vi "Z900_navX_ProcessingLoop.vi"(11 "navX Device":T1={"Interface"={"Protocol"=enum."SERIAL", "Update Rate (4Hz-60Hz)"=4, "navX Open TypeDef"=variant}, "Notify Packet"=refnum, "Loop VI Refnum"=refnum} {"Interface"."Update Rate (4Hz-60Hz)" min=4 max=60 step=1}) -> (2 "Local Registry":u8[](array[numeric]))   [LabVIEW 2014, in "navX Library v2.lvlib"]
uses:
  navX Library v2.lvlib
  TypeDefs/Z900_navX_DeviceTypeDef.ctl
  TypeDefs/Z900_navX_ProtocolTypeDef.ctl
  TypeDefs/Z900_navX_NotifyPacketTypeDef.ctl
  TypeDefs/Z900_navX_ActionTypeDef.ctl
  <vilib>/Platform/TimedLoop/XDataNode/timing_clust.ctl
  <vilib>/Platform/TimedLoop/XDataNode/nitl_modes.ctl
  <vilib>/Platform/TimedLoop/XDataNode/wakeup.ctl
  <vilib>/Rock Robotics/SystemInterfaces/Utilities/FPGA_UtilitiesRead LocalTime.vi
  <vilib>/platform/TimedLoop/XDataNode/XDataNode.xnode
  <vilib>/Platform/TimedLoop/XDataNode/XDNodeRunTimeDep.lvlib
panel:
  in  "Halt":bool
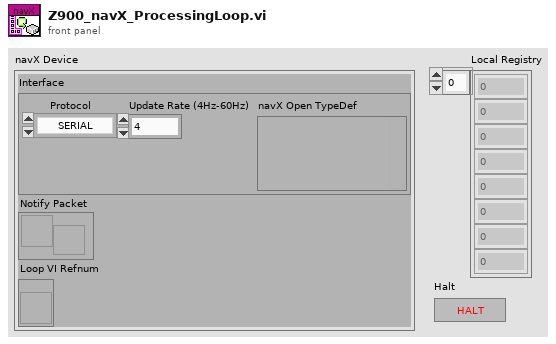
[diagram p1: front panel]
types:
  T1 = typedef "navX Library v2.lvlib/Z900_navX_DeviceTypeDef.ctl" = cluster{"Interface":cluster{"Protocol":T2, "Update Rate (4Hz-60Hz)":u8, "navX Open TypeDef":variant}, "Notify Packet":refnum<notifier>, "Loop VI Refnum":refnum<vi>}
  T2 = typedef "navX Library v2.lvlib/Z900_navX_ProtocolTypeDef.ctl" = enum16{"SERIAL", "I2C", "SPI"}
  T3 = cluster{"Last Valid FPGA Time":dbl, "Error Count":i32, "Initialized":bool}
  T4 = typedef "navX Library v2.lvlib/Z900_navX_InterfaceTypeDef.ctl" = cluster{"SerialPortRef":T5, "I2CDevRef":T6, "SPIDevRef":T9}
  T5 = typedef "WPI_SerialPortRef.ctl" = cluster{"DevStatus":errorcluster, "Serial Port Name":refnum<visa-resource-name>}
  T6 = typedef "WPI_I2CDevRef.ctl" = cluster{"DevStatus":errorcluster, "Controller":T7, "Device Address":u8, "Handle":i32, "I2C Bus":T8}
  T7 = typedef "FPGA_TypedefDigitalModule.ctl" = enum16{"Controller 1"}
  T8 = typedef "i2c_bus.ctl" = enum16{"I2C On-Board", "I2C MXP", "Invalid"}
  T9 = typedef "WPI_SPIDevRef.ctl" = cluster{"DevStatus":errorcluster, "Handle":i32, "Controller":T7, "SPI Bus":T10}
  T10 = typedef "spi_bus.ctl" = enum16{"SPI On-Board, CS0", "SPI On-Board, CS1", "SPI On-Board, CS2", "SPI On-Board, CS3", "SPI MXP", "Invalid"}
  T11 = typedef "XDNodeRunTimeDep.lvlib/timing_clust.ctl" = cluster{"Expected End [f-1]":u64, "Actual End [f-1]":u64, "Finished Late? [f-1]":bool, "Expected End [i-1]":u64, "Actual End [i-1]":u64, "Finished Late? [i-1]":bool, "Expected Start [i]":u64, "Actual Start [i]":u64, "Expected Start [f]":u64, "Actual Start [f]":u64, "Source Name":string, "Structure Name":string, "Period":i64, "Deadline":i64, "Offset":i64, "Start":i64, "Priority":i32, "Timeout":i32, "Mode":T12, "Wakeup Reason":T13, "Error":errorcluster, "Source Type":string, "Secondary Source Type":string, "Global End Time":u64, "Global Start Time":u64, "Frame Duration":u64, "Iteration Duration":u64, "Assigned CPU":i32, "I/O Scan Engine Mode":u32}
  T12 = typedef "XDNodeRunTimeDep.lvlib/nitl_modes.ctl" = enum32{"No Change", "Process missed periods, maintain original phase", "Discard missed periods, maintain original phase", "Process missed periods, ignore original phase", "Discard missed periods, ignore original phase"}
  T13 = typedef "XDNodeRunTimeDep.lvlib/wakeup.ctl" = enum32{"Normal", "Aborted", "Asynchronous wakeup", "Timing source error", "Timed loop error", "Timeout"}
  T14 = typedef "navX Library v2.lvlib/Z900_navX_NotifyPacketTypeDef.ctl" = cluster{"navX Action":T15, "Data":variant}
  T15 = typedef "navX Library v2.lvlib/Z900_navX_ActionTypeDef.ctl" = enum16{"None", "Halt", "Reboot Detected", "Zero-Yaw"}
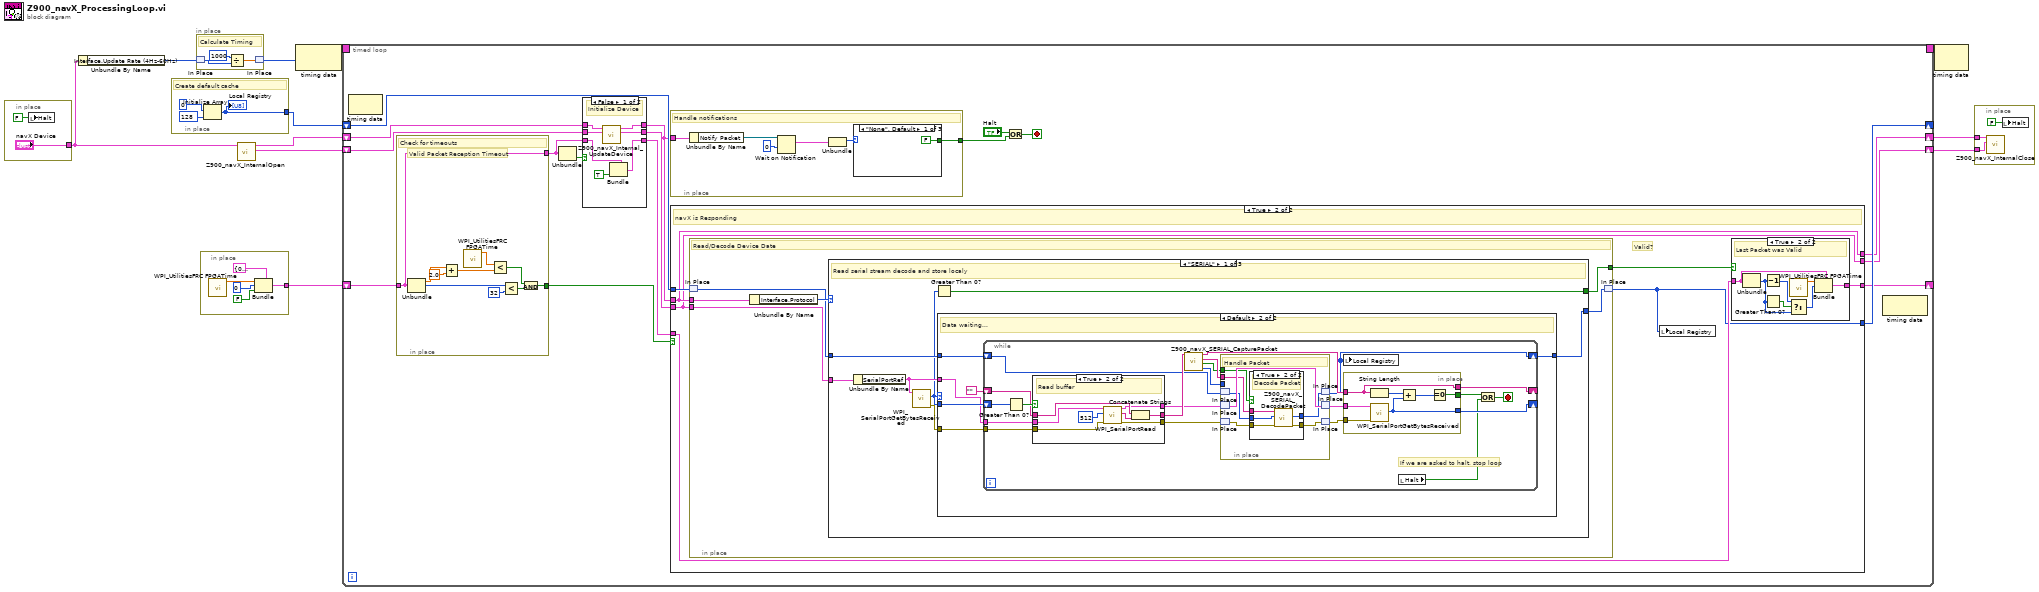
[diagram p0: block diagram]
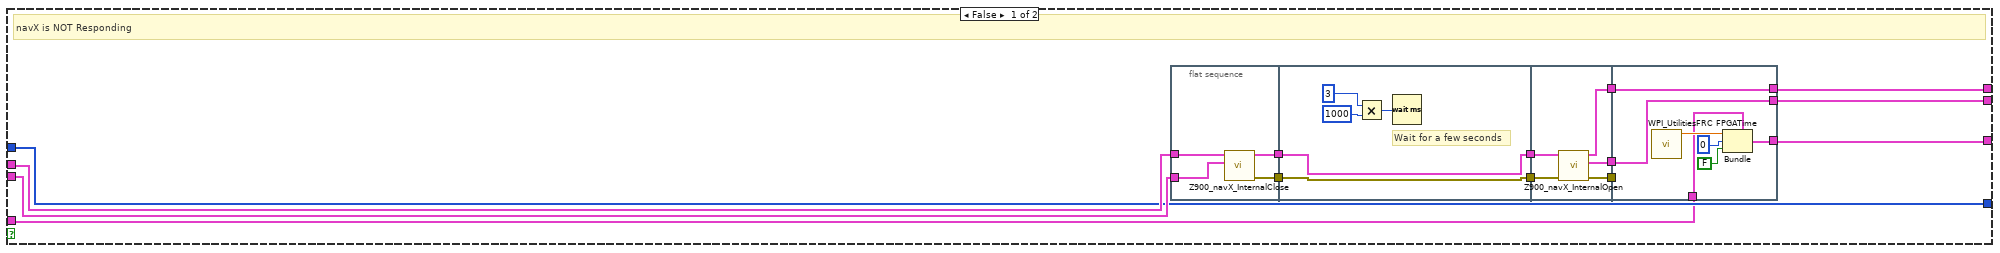
[diagram p3: hidden frame]
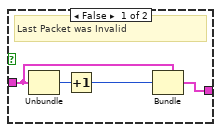
[diagram p4: hidden frame]
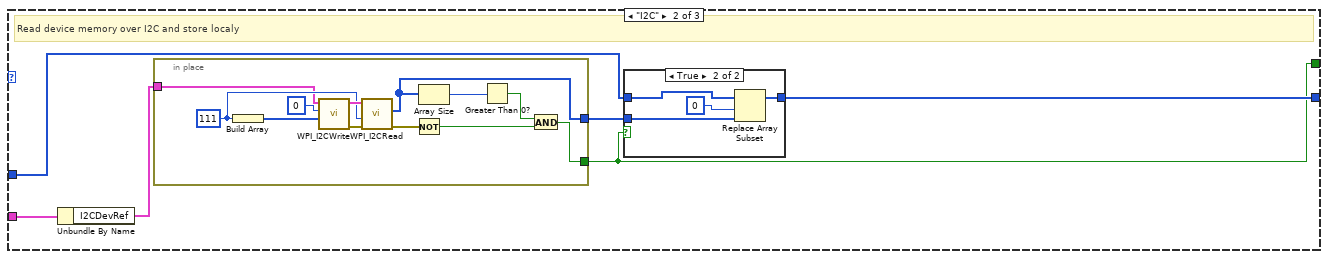
[diagram p8: hidden frame]
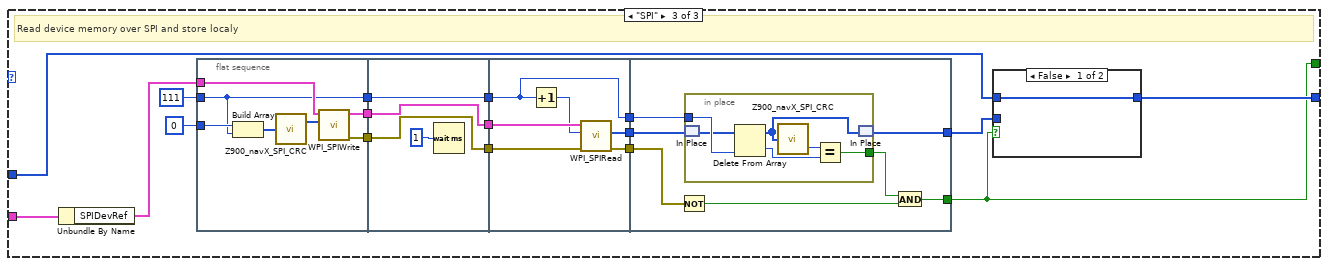
[diagram p10: hidden frame]
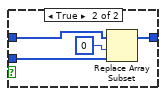
[diagram p11: hidden frame]
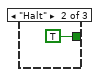
[diagram p12: hidden frame]
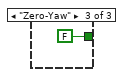
[diagram p13: hidden frame]
diagram:
  n1 = in-place {
    in-place-border: ["navX Device"] -> w4
    n2 = local write "Halt"(FALSE ("Halt")) -> ()
  }
  n3 = Unbundle By Name(w4) -> ("Interface.Update Rate (4Hz-60Hz)"=w8:u8)
  n4 = in-place {
    in-place-border: [w14] -> w7
    # "Create default cache"
    n5 = Initialize Array(u8 0 ("Received Data"), 128 ("hex")) -> (w14:u8[])
    "Local Registry" <- w14
  }
  n6 = in-place {
    # "Calculate Timing"
    n7 = in-place-match #1(w8) -> (w18:u8)
    n8 = Divide(x=1000, y=w18) -> (x/y=w17:dbl)
    n9 = in-place-match #1(w17) -> (w9:u8)
  }
  n10 = in-place {
    in-place-border: [w22] -> w2
    n11 = call <vilib>:"WPI_UtilitiesFRC FPGATime.vi"() -> ("FPGA Time"=w23:dbl)  [unwired: 10 in, 1 out]
    n12 = Bundle(cluster=T3 {"Last Valid FPGA Time"=0.0, "Error Count"=0, "Initialized"=FALSE}, "Last Valid FPGA Time"=w23, "Error Count"=0, "Initialized"=FALSE) -> (w22:T3)
  }
  n13 = call "Z900_navX_InternalOpen.vi"("navX Device"=w4) -> ("Interface TypeDefs"=w3:T4, "navX Device"=w1:T1)  [unwired: 8 in, 1 out]
  n14 = node-c288(w9) -> (w11:T11)
  n15 = timed-loop {
    timing: w11 -> [_]
    timing-out: [_] -> w10
    shift-right: [w40] -> _
    shift-left: w7 -> [w41]
    shift-right: [w34] -> w6
    shift-left: w1 -> [w31]
    shift-right: [w33] -> w5
    shift-left: w3 -> [w30]
    shift-right: [w39] -> _
    shift-left: w2 -> [w25]
    stop <- w36 stop-if-true
    n16 = node-c288() -> ()  [unwired: 1 in, 1 out]
    n17 = in-place {
      in-place-border: w25 -> [w52]
      in-place-border: [w53] -> w35
      in-place-border: [w52] -> w27
      # "Valid Packet Reception Timeout"
      # "Check for timeouts"
      n18 = Unbundle(w52) -> ("Last Valid FPGA Time"=w61:dbl, "Error Count"=w57:i32)  [unwired: 1 out]
      n19 = Add(x=w61, y=2.0) -> (x+y=w59:dbl)
      n20 = call <vilib>:"WPI_UtilitiesFRC FPGATime.vi"() -> ("FPGA Time"=w58:dbl)  [unwired: 10 in, 1 out]
      n21 = Less?(x=w58, y=w59) -> (x < y?=w55:bool)
      n22 = Less?(x=w57, y=32) -> (x < y?=w54:bool)
      n23 = And(x=w55, y=w54) -> (x .and. y?=w53:bool)
    }
    n24 = Unbundle(w27) -> ("Initialized"=w32:bool)  [unwired: 2 out]
    n25 = case shown="False" w32 {
      tunnel: w27 -> [w48 w51]
      tunnel: [w46 w51] -> w26
      tunnel: w31 -> [w45 w50]
      tunnel: w30 -> [w44 w49]
      tunnel: [w43 w50] -> w28
      tunnel: [w42 w49] -> w29
      frame False {
        # "Initialize Device"
        n26 = call "Z900_navX_Internal_UpdateDevice.vi"("Interface TypeDefs"=w44, "navX Device"=w45) -> ("Interface TypeDefs"=w42:T4, "navX Device"=w43:T1)  [unwired: 7 in, 1 out]
        n27 = Bundle(cluster=w48, "Initialized"=TRUE) -> (w46:T3)  [unwired: 2 in]
      }
      frame True {
      }
    }
    n28 = in-place {
      in-place-border: [w266] -> w38
      in-place-border: w28 -> [w265]
      # "Handle notifications"
      n29 = Unbundle By Name(w265) -> ("Notify Packet"=w264:refnum<notifier>)
      n30 = Wait on Notification(notifier=w264, timeout in ms (-1)=0) -> (notification=w268:T14)  [unwired: 2 in, 3 out]
      n31 = Unbundle(w268) -> ("navX Action"=w267:T15)  [unwired: 1 out]
      n32 = case shown="\"None\", Default" w267 {
        tunnel: [FALSE TRUE FALSE] -> w266
        frame "None", Default {
        }
        frame "Halt" {
        }
        frame "Zero-Yaw" {
        }
      }
    }
    n33 = case shown="True" w35 {
      tunnel: w41 -> [w73 w103]
      tunnel: w29 -> [w74 w100]
      tunnel: [w73 w97] -> w40
      tunnel: w26 -> [w63 w99]
      tunnel: [w62 w98] -> w39
      tunnel: w28 -> [w75 w101]
      tunnel: [w68 w101] -> w34
      tunnel: [w67 w100] -> w33
      frame False {
        # "navX is NOT Responding"
        n34 = flat-sequence {
          tunnel: w75 -> [w79]
          tunnel: w74 -> [w78]
          tunnel: [w77] -> w72
          tunnel: [w76] -> w71
          tunnel: w72 -> [w84]
          tunnel: w71 -> [w83]
          tunnel: [w84] -> w70
          tunnel: [w83] -> w69
          tunnel: w70 -> [w87]
          tunnel: w69 -> [w88]
          tunnel: [w89] -> w66
          tunnel: [w86] -> w65
          tunnel: [w85] -> w64
          tunnel: [w95] -> w67
          tunnel: [w96] -> w68
          tunnel: w66 -> [w96]
          tunnel: w65 -> [w95]
          tunnel: w64 -> [_]
          tunnel: w63 -> [w92]
          tunnel: [w91] -> w62
          frame #0 {
            n35 = call "Z900_navX_InternalClose.vi"("Interface TypeDefs"=w78, "navX Device"=w79) -> ("error out"=w77:errorcluster, "navX Device"=w76:T1)  [unwired: 8 in]
          }
          frame #1 {
            # "Wait for a few seconds"
            n36 = Multiply(x=u32 3 ("milliseconds to wait"), y=u32 1000) -> (x*y=w81:u32)
            n37 = Wait (ms)(milliseconds to wait=w81) -> ()  [unwired: 1 out]
          }
          frame #2 {
            n38 = call "Z900_navX_InternalOpen.vi"("error in"=w87, "navX Device"=w88) -> ("error out"=w85:errorcluster, "Interface TypeDefs"=w86:T4, "navX Device"=w89:T1)  [unwired: 7 in]
          }
          frame #3 {
            n39 = call <vilib>:"WPI_UtilitiesFRC FPGATime.vi"() -> ("FPGA Time"=w93:dbl)  [unwired: 10 in, 1 out]
            n40 = Bundle(cluster=w92, "Last Valid FPGA Time"=w93, "Error Count"=0, "Initialized"=FALSE) -> (w91:T3)
          }
        }
      }
      frame True {
        # "Valid?"
        # "navX is Responding"
        n41 = in-place {
          in-place-border: w101 -> [w115]
          in-place-border: w100 -> [w119]
          in-place-border: [w117] -> w102
          # "Read/Decode Device Date"
          n42 = in-place-match #2(w103) -> (w118:u8[])
          n43 = Unbundle By Name(w115) -> ("Interface.Protocol"=w120:T2)
          n44 = case shown="\"SERIAL\"" w120 {
            tunnel: [w125 w190 w218] -> w116
            tunnel: w118 -> [w126 w192 w227]
            tunnel: w119 -> [w127 w193 w226]
            tunnel: [w122 w189 w215] -> w117
            frame "SERIAL" {
              # "Read serial stream decode and store localy"
              n45 = Unbundle By Name(w127) -> ("SerialPortRef"=w123:T5)
              n46 = call <vilib>:"WPI_SerialPortGetBytesReceived.vi"("SerialPortRef"=w123) -> ("error out"=w124:errorcluster, "Bytes at Port"=w121:u32)  [unwired: 8 in, 1 out]
              n47 = Greater Than 0?(x=w121) -> (x > 0?=w122:bool)
              n48 = case shown="Default" w121 {
                tunnel: [w128 w134] -> w125
                tunnel: w126 -> [w128 w133]
                tunnel: w121 -> [_ w132]
                tunnel: w123 -> [_ w130]
                tunnel: w124 -> [_ w129]
                frame 0 {
                }
                frame Default {
                  # "Data waiting..."
                  n49 = while {
                    shift-right: [w135] -> w134
                    shift-left: w133 -> [w144]
                    shift-right: [w148] -> _
                    shift-left: w132 -> [w155]
                    shift-right: [w147] -> _
                    shift-left: "" -> [w153]
                    tunnel: w130 -> [w152]
                    tunnel: w129 -> [w151]
                    stop <- w138 stop-if-true
                    # "If we are asked to halt, stop loop"
                    n50 = Greater Than 0?(x=w155) -> (x > 0?=w154:bool)
                    n51 = case shown="True" w154 {
                      tunnel: w153 -> [w179 w187]
                      tunnel: w152 -> [w178 w186]
                      tunnel: w151 -> [w177 w183]
                      tunnel: [w179 w182] -> w150
                      tunnel: [w178 w181] -> w143
                      tunnel: [w177 w180] -> w142
                      frame False {
                        # "Pass existing buffer"
                      }
                      frame True {
                        # "Read buffer"
                        n52 = call <vilib>:"WPI_SerialPortRead.vi"("error in (no error)"=w183, "Num Bytes to Read"=u32 512, "SerialPortRef"=w186) -> ("error out"=w180:errorcluster, "Buffer"=w185:string, "SerialPortRef"=w181:T5)  [unwired: 6 in]
                        n53 = Concatenate Strings(w187, w185) -> (w182:string)
                      }
                    }
                    n54 = call "Z900_navX_SERIAL_CapturePacket.vi"("Buffer"=w150) -> ("Packet Size"=w145:i32, "Packet Located"=w136:bool, "Packet"=w146:string, "Buffer"=w149:string)  [unwired: 7 in]
                    n55 = in-place {
                      in-place-border: w146 -> [w160]
                      in-place-border: w136 -> [w161]
                      in-place-border: w145 -> [_]
                      # "Handle Packet"
                      n56 = in-place-match #3(w144) -> (w158:u8[])
                      n57 = in-place-match #4(w143) -> (w162:T5)
                      n58 = in-place-match #5(w142) -> (w157:errorcluster)
                      n59 = case shown="True" w161 {
                        tunnel: w160 -> [_ w169]
                        tunnel: [w164 w167] -> w159
                        tunnel: w158 -> [w164 w168]
                        tunnel: w157 -> [w163 w166]
                        tunnel: [w163 w165] -> w156
                        frame False {
                          # "No Packet"
                        }
                        frame True {
                          # "Decode Packet"
                          n60 = call "Z900_navX_SERIAL_DecodePacket.vi"("error in (no error)"=w166, "Data"=w168, "Packet"=w169) -> ("error out"=w165:errorcluster, "Data"=w167:u8[])  [unwired: 6 in, 1 out]
                        }
                      }
                      n61 = in-place-match #3(w159) -> (w135:u8[])
                      n62 = in-place-match #4(w162) -> (w140:T5)
                      n63 = in-place-match #5(w156) -> (w141:errorcluster)
                    }
                    n64 = local write "Local Registry"(w135) -> ()
                    n65 = in-place {
                      in-place-border: w140 -> [w176]
                      in-place-border: w141 -> [w175]
                      in-place-border: w149 -> [w170]
                      in-place-border: [w172] -> w139
                      in-place-border: [w171] -> w148
                      in-place-border: [w170] -> w147
                      n66 = String Length(string=w170) -> (length=w173:i32)
                      n67 = call <vilib>:"WPI_SerialPortGetBytesReceived.vi"("error in (no error)"=w175, "SerialPortRef"=w176) -> ("Bytes at Port"=w171:u32)  [unwired: 7 in, 2 out]
                      n68 = Add(x=w173, y=w171) -> (x+y=w174:u32)
                      n69 = Equal To 0?(x=w174) -> (x = 0?=w172:bool)
                    }
                    n70 = local read "Halt"() -> (w137:bool)
                    n71 = Or(x=w139, y=w137) -> (x .or. y?=w138:bool)
                  }
                }
              }
            }
            frame "I2C" {
              # "Read device memory over I2C and store localy"
              n72 = Unbundle By Name(w193) -> ("I2CDevRef"=w188:T6)
              n73 = in-place {
                in-place-border: [w197] -> w191
                in-place-border: [w196] -> w189
                in-place-border: w188 -> [w194]
                w202 = u8 111 ("hex")
                n74 = Build Array(w202) -> (w205:u8[])
                n75 = call <vilib>:"WPI_I2CWrite.vi"("I2CDataToSend"=w205, "I2CRegister"=u8 0 ("hex"), "I2CDevRef"=w194) -> ("error out"=w204:errorcluster, "I2CDevRef"=w203:T6)  [unwired: 7 in]
                n76 = call <vilib>:"WPI_I2CRead.vi"("error in (no error)"=w204, "I2CBytesToRead"=w202, "I2CDevRef"=w203) -> ("error out"=w198:errorcluster, "Data Out"=w197:u8[])  [unwired: 6 in, 1 out]
                n77 = Not(x=w198) -> (.not. x?=w195:bool)
                n78 = Array Size(array=w197) -> (size(s)=w200:i32)
                n79 = Greater Than 0?(x=w200) -> (x > 0?=w199:bool)
                n80 = And(x=w199, y=w195) -> (x .and. y?=w196:bool)
              }
              n81 = case shown="True" w189 {
                tunnel: w192 -> [w206 w210]
                tunnel: [w206 w209] -> w190
                tunnel: w191 -> [_ w208]
                frame False {
                }
                frame True {
                  n82 = Replace Array Subset(array=w210, new element=w208, index=u8 0 ("hex")) -> (w209:u8[])
                }
              }
            }
            frame "SPI" {
              # "Read device memory over SPI and store localy"
              n83 = Unbundle By Name(w226) -> ("SPIDevRef"=w211:T9)
              n84 = flat-sequence {
                tunnel: u8 0 ("hex") -> [w239]
                tunnel: u8 111 ("hex") -> [w234]
                tunnel: w211 -> [w236]
                tunnel: [w235] -> w224
                tunnel: [w234] -> w221
                tunnel: [w233] -> w214
                tunnel: w224 -> [w242]
                tunnel: [w242] -> w223
                tunnel: [w241] -> w222
                tunnel: w221 -> [w241]
                tunnel: w214 -> [w240]
                tunnel: [w240] -> w213
                tunnel: w223 -> [w249]
                tunnel: w222 -> [w246]
                tunnel: [w247] -> w220
                tunnel: [w246] -> w219
                tunnel: w213 -> [w245]
                tunnel: [w244] -> w212
                tunnel: w220 -> [w252]
                tunnel: w219 -> [w256]
                tunnel: [w253] -> w215
                tunnel: [w251] -> w217
                tunnel: w212 -> [w255]
                frame #0 {
                  n85 = Build Array(w239, w234) -> (w238:u8[])
                  n86 = call "Z900_navX_SPI_CRC.vi"("Message"=w238) -> ("Message with CRC"=w237:u8[])  [unwired: 1 out]
                  n87 = call <vilib>:"WPI_SPIWrite.vi"("Data To Send"=w237, "SPIDevRef"=w236) -> ("error out"=w233:errorcluster, "SPIDevRef"=w235:T9)  [unwired: 7 in, 1 out]
                }
                frame #1 {
                  n88 = Wait (ms)(milliseconds to wait=u32 1) -> ()  [unwired: 1 out]
                }
                frame #2 {
                  n89 = Increment(x=w246) -> (x+1=w248:u8)
                  n90 = call <vilib>:"WPI_SPIRead.vi"("error in (no error)"=w245, "Num to Read"=w248, "SPIDevRef"=w249) -> ("error out"=w244:errorcluster, "Received Data"=w247:u8[])  [unwired: 6 in, 1 out]
                }
                frame #3 {
                  n91 = Not(x=w255) -> (.not. x?=w250:bool)
                  n92 = in-place {
                    in-place-border: w256 -> [w262]
                    in-place-border: [w259] -> w254
                    n93 = in-place-match #6(w252) -> (w258:u8[])
                    n94 = Delete From Array(array=w258, index=w262) -> (deleted portion=w261:u8, array with subset deleted=w257:u8[])  [unwired: 1 in]
                    n95 = call "Z900_navX_SPI_CRC.vi"("Message"=w257) -> ("CRC"=w260:u8)  [unwired: 1 out]
                    n96 = Equal?(x=w260, y=w261) -> (x = y?=w259:bool)
                    n97 = in-place-match #6(w257) -> (w251:u8[])
                  }
                  n98 = And(x=w254, y=w250) -> (x .and. y?=w253:bool)
                }
              }
              n99 = case shown="False" w215 {
                tunnel: w227 -> [w228 w232]
                tunnel: [w228 w231] -> w218
                tunnel: w217 -> [_ w230]
                frame False {
                }
                frame True {
                  n100 = Replace Array Subset(array=w232, new element=w230, index=u8 0 ("hex")) -> (w231:u8[])
                }
              }
            }
          }
          n101 = in-place-match #2(w116) -> (w97:u8[])
        }
        n102 = local write "Local Registry"(w97) -> ()
        n103 = case shown="True" w102 {
          tunnel: [w104 w113] -> w98
          tunnel: w99 -> [w105 w108]
          frame False {
            # "Last Packet was Invalid"
            n104 = Unbundle(w105) -> ("Error Count"=w106:i32)  [unwired: 2 out]
            n105 = Increment(x=w106) -> (x+1=w107:i32)
            n106 = Bundle(cluster=w105, "Error Count"=w107) -> (w104:T3)  [unwired: 2 in]
          }
          frame True {
            # "Last Packet was Valid"
            n107 = Unbundle(w108) -> ("Error Count"=w109:i32)  [unwired: 2 out]
            n108 = Decrement(x=w109) -> (x-1=w111:i32)
            n109 = Greater Than 0?(x=w109) -> (x > 0?=w112:bool)
            n110 = Select(t=w111, s=w112, f=w109) -> (s? t:f=w110:i32)
            n111 = call <vilib>:"WPI_UtilitiesFRC FPGATime.vi"() -> ("FPGA Time"=w114:dbl)  [unwired: 10 in, 1 out]
            n112 = Bundle(cluster=w108, "Last Valid FPGA Time"=w114, "Error Count"=w110) -> (w113:T3)  [unwired: 1 in]
          }
        }
      }
    }
    n113 = Or(x="Halt", y=w38) -> (x .or. y?=w36:bool)
    n114 = node-c288() -> ()  [unwired: 1 in, 1 out]
  }
  n115 = node-c288(w10) -> ()  [unwired: 1 out]
  n116 = in-place {
    in-place-border: w6 -> [w276]
    in-place-border: w5 -> [w275]
    n117 = call "Z900_navX_InternalClose.vi"("Interface TypeDefs"=w275, "navX Device"=w276) -> ()  [unwired: 8 in, 2 out]
    n118 = local write "Halt"(FALSE ("Halt")) -> ()
  }
